vi "Dashboard Main.vi"() -> ()   [LabVIEW 2015]
uses:
  <vilib>/event_ctls.llb/eventvkey.ctl
  <vilib>/Utility/config.llb/NI_LVConfig.lvlib
  <vilib>/Rock Robotics/WPI/Dashboard/WPI_DashboardLogging Global.vi
  <vilib>/Utility/config.llb/Write Key (String).vi
  <vilib>/Utility/config.llb/Write Key (I32).vi
  TargetType.ctl
  <vilib>/Rock Robotics/WPI/Camera/WPI_CameraExposure Values.ctl
  <vilib>/Rock Robotics/WPI/Camera/WPI_CameraWhite Balance Values.ctl
panel:
  out "Image Message":string="Timeout in Camera Communications"
  in  "Rec Mode":enum32{"Stop", "Record", "Playback"}(radio)
  in  "Dashboard Tab":T1(tab)
  in  "Camera Settings":T2={"Frame Rate"=30, "Compression"=30, "Size"=1} {"Frame Rate" scale=1.0..30.0; "Size" items=["640x480", "320x240", "160x120"]}
  out "MotorSliders R":cluster{"MotorSlide1":dbl, "MotorSlide2":dbl} {"MotorSlide2" scale=-1.0..1.0 scale format="%#_2e"; "MotorSlide1" scale=-1.0..1.0 scale format="%#_2e"}
  out "MotorChart R":cluster{"Numeric":dbl, "Numeric":dbl}(graph)
  out "MotorSliders L":T3 {"MotorSlide4 2" scale=0.0..14.0 scale format="%#_2e"; "MotorSlide2" scale=-1.0..1.0 scale format="%#_2e"; "MotorSlide1" scale=-1.0..1.0 scale format="%#_2e"}
  out "MotorChart L":T4(graph)
  out "JS1 Z":dbl(slide) scale=-1.0..1.0 scale format="%#_2e"
  out "Joystick 1":cluster{"X":dbl, "Y":dbl}[](graph)
  out "JS Buttons 1":T5
  out "JS2 Z":dbl(slide) scale=-1.0..1.0 scale format="%#_2e"
  out "Joystick 2":cluster{"X":dbl, "Y":dbl}[](graph)
  out "JS Buttons 2":T5
  out "Mode":T6(ring)=enum."Auto Disabled"
  out "Camera IP":string
  in  "DB Camera Config":bool
  out "fps":dbl format="%#.1g"
  out "Mbps":dbl format="%#.1g"
  out "Mbps 2":bool
  out "LED 1":bool
  in  "Brightness":dbl(slide) scale=0.0..100.0
  in  "Color Level":dbl(slide) scale=0.0..100.0
  in  "Sharpness":dbl(slide) scale=0.0..100.0
  in  "Exposure":T7=enum."Hold current"
  in  "White Balance":T8
  in  "Move":T9(ring)=enum."Rook"
  in  "Score Limit":dbl=70.0
  in  "Color Components":T10={"Hue"={110.0, 142.0}, "Sat"={138.0, 255.0}, "Val"={139.0, 198.0}} {"Val" scale=0.0..255.0; "Sat" scale=0.0..255.0; "Hue" scale=0.0..255.0 scale format="%#_3g"}
  in  "Checkbox 2":bool
  in  "Checkbox 1":bool
  in  "Test Slider":dbl(slide) scale=0.0..100.0 scale format="%#_3g"
  in  "On/Off":bool caption="Solenoid"
  in  "Test Name":u16(ring) items=["Select the test to run...", "Example Test", "-------------------------------", "List of tests is built in robot code.", "Replace with your own automated tests."]
  in  "Test Tree":string(tree)
  in  "Motor":cluster{"Value":dbl, "Enable":bool} {"Value" scale=-1.0..1.0 scale format="%#_3g"}
  out "Progress":T11 {"Test Progress" scale=0.0..100.0}
  in  "Rev/Fwd":cluster{"Forward":bool, "Reverse":bool}
  in  "Test Ring":u16(ring) items=["Auto", "Fixed indoor", "Fixed outdoor 1", "Fixed outdoor 2", "Fixed fluorescent 1", "Fixed fluorescent 2", "Hold current"]
  in  "Listbox":i32(listbox)
  out "Tree":string(tree)
  out "Camera Image":T12(plugin-control)
  in  "Enable":bool=TRUE
  # "Left"
  # "Front"
  # "Right"
  # "Battery"
  # "This tab is a great place for autonomous settings and validation.\nCustomize by placing controls and indicators here and name to\nmatch Dashboard Variables on robot."
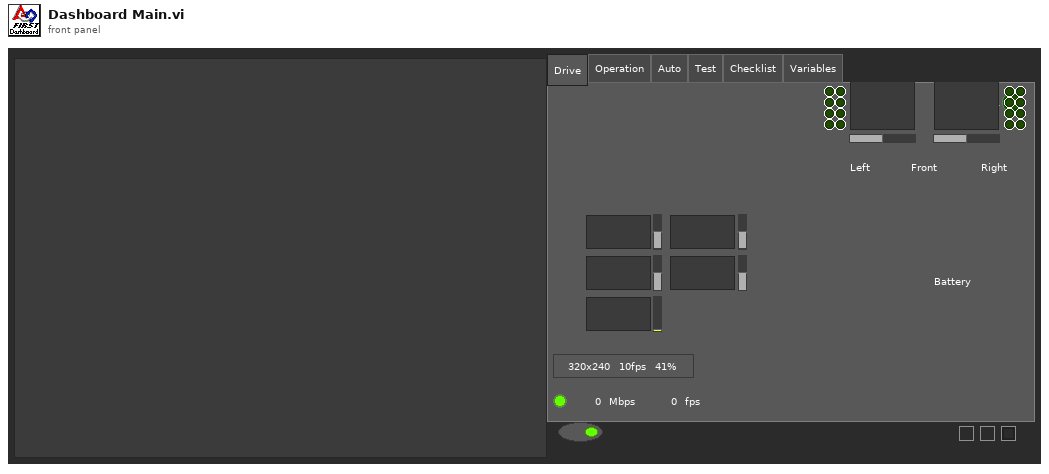
[diagram p1: front panel]
types:
  T1 = enum32{"Drive", "Operation", "Auto", "Test", "Checklist", "Variables"}
  T2 = cluster{"Frame Rate":i32, "Compression":i32, "Size":u16}
  T3 = cluster{"MotorSlide1":dbl, "MotorSlide2":dbl, "MotorSlide4 2":dbl}
  T4 = cluster{"Numeric":dbl, "Numeric":dbl, "Battery":sgl}
  T5 = cluster{bool, bool, bool, bool, bool, bool, bool, bool, bool, bool, bool, bool}
  T6 = enum8{"Tele-Op Disabled", "Tele-Op Enabled", "Auto Disabled", "Auto Enabled", "Test Disabled", "Test Enabled", ""}
  T7 = typedef "WPI_CameraExposure Values.ctl" = enum16{"Auto", "Flicker-free 50 Hz", "Flicker-free 60 Hz", "Hold current", "Custom"}
  T8 = typedef "WPI_CameraWhite Balance Values.ctl" = enum16{"Auto", "Fixed indoor", "Fixed outdoor 1", "Fixed outdoor 2", "Fixed fluorescent 1", "Fixed fluorescent 2", "Hold current", "Custom"}
  T9 = enum16{"Queen", "King", "Rook", "Knight", "Pawn"}
  T10 = cluster{"Hue":cluster{dbl, dbl}, "Sat":cluster{dbl, dbl}, "Val":cluster{dbl, dbl}}
  T11 = cluster{"Test Progress":u8, "Test Progress Text":string}
  T12 = typedef "IMAQ Image.ctl" = refnum<image>
  T13 = typedef "Image Type" = u32
  T14 = typedef "TargetType.ctl" = enum16{"Not Hot", "Hot"}
  T15 = cluster{"Horizontal":bool, "Aspect Score":dbl, "Rect Score":dbl, cluster{"Left":dbl, "Top":dbl, "Right":dbl, "Bottom":dbl}, "Equiv H":dbl, "Equiv V":dbl}[]
  T16 = cluster{"Scores":cluster{"Total":dbl, "Left":dbl, "Right":dbl, "Ratio":dbl, "Vertical":dbl, "index":i32, "State":T14}, "Verticals":cluster{"Horizontal?":bool, "Aspect Score":dbl, "Rect Score":dbl, cluster{"Left":dbl, "Top":dbl, "Right":dbl, "Bottom":dbl}, "Equiv H":dbl, "Equiv V":dbl}, "Horizontals":cluster{"Horizontal?":bool, "Aspect Score":dbl, "Rect Score":dbl, cluster{"Left":dbl, "Top":dbl, "Right":dbl, "Bottom":dbl}, "Equiv H":dbl, "Equiv V":dbl}, "Validated":bool}[]
  T17 = cluster{"Distance (ft)":dbl, "Target Center (-1 to 1)":cluster{"X":dbl, "Y":dbl}, "Left":bool, "State":T14, "Angle":dbl}[]
  T18 = cluster{cluster{dbl, dbl}, cluster{dbl, dbl}, cluster{dbl, dbl}}
  T19 = cluster{"Distance (ft)":dbl, "Target Center (-1 to 1)":cluster{"X":dbl, "Y":dbl}, "Left":bool, "State":T14, "Angle":dbl}
  T20 = cluster{"Digital Inputs":bool[], "Digital Outputs":bool[]}
  T21 = cluster{"Competition mode":bool, "Robot Link":bool, "Autonomous":bool, "Enabled":bool, "E-Stop":bool, "Simulated":bool, "TestMode":bool, "Docked Window":bool}
  T22 = cluster{"Boolean Array[0]":bool, "Boolean Array[1]":bool, "Boolean Array[2]":bool, "Boolean Array[3]":bool, "Boolean Array[4]":bool, "Boolean Array[5]":bool, "Boolean Array[6]":bool, "Boolean Array[7]":bool, "Boolean Array[8]":bool, "Boolean Array[9]":bool, "Boolean Array[10]":bool, "Boolean Array[11]":bool}
  T23 = typedef "NI_LVConfig.lvlib/Config Data RefNum.ctl" = refnum<k1>
  T24 = typedef "eventvkey.ctl" = enum16{"ASCII", "Enter", "Return", "Shift", "Ctrl", "Alt", "Cmd", "Opt", "Caps", "NumLock", "Clear", "Break", "Up", "Down", "Left", "Right", "Insert", "Delete", "Home", "End", "PageUp", "PageDown", "Escape", "Help", "Pause", "ScrollLock", "F1", "F2", "F3", "F4", "F5", "F6", "F7", "F8", "F9", "F10", "F11", "F12", "F13", "F14", "F15", "F16", "F17", "F18", "F19", "F20", "F21", "F22", "F23", "F24", "Play", "VolumeUp", "VolumeDown", "Mute", "Two Byte Char"}
  T25 = cluster{"Image Size":bool, "Image Type":bool, "Pixel Value":bool, "ROI Information":bool, "Zoom Factor":bool}
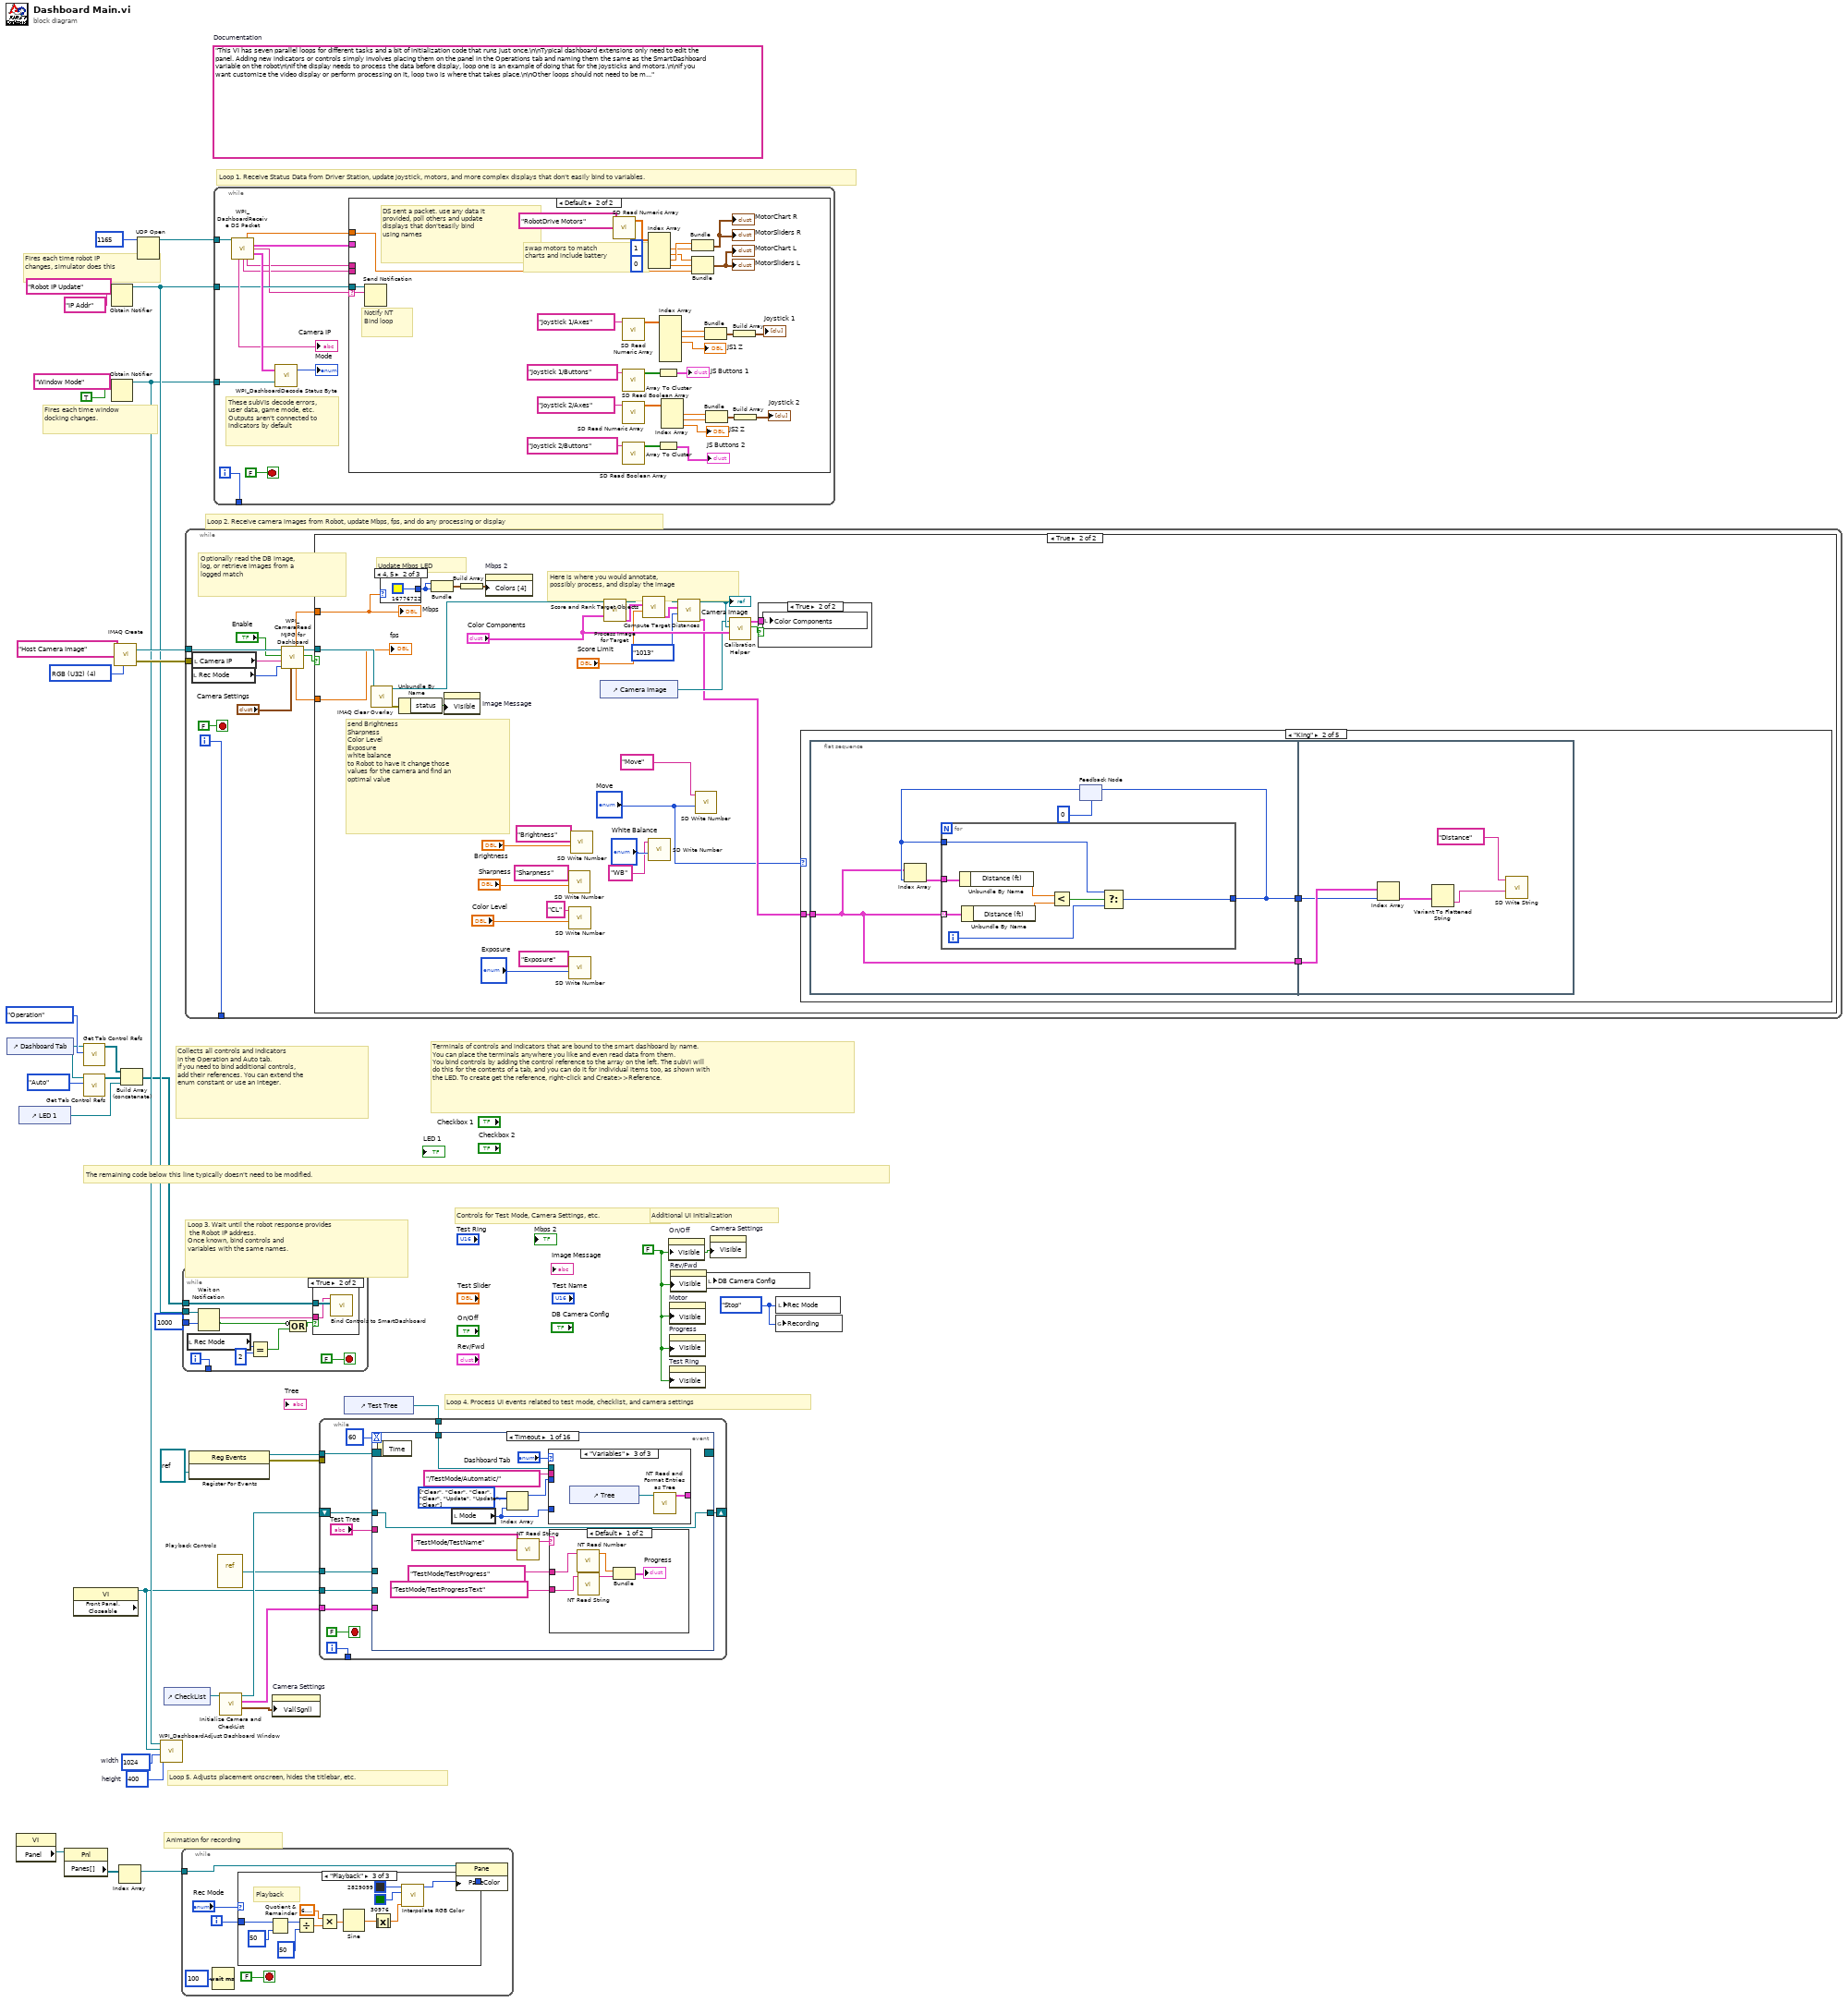
[diagram p0: block diagram]
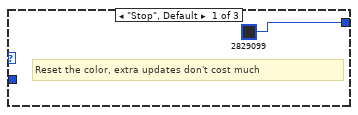
[diagram p2: hidden frame]
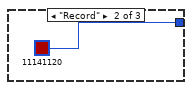
[diagram p3: hidden frame]
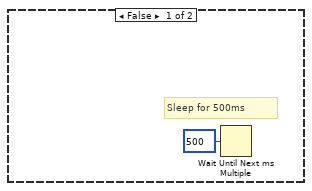
[diagram p5: hidden frame]
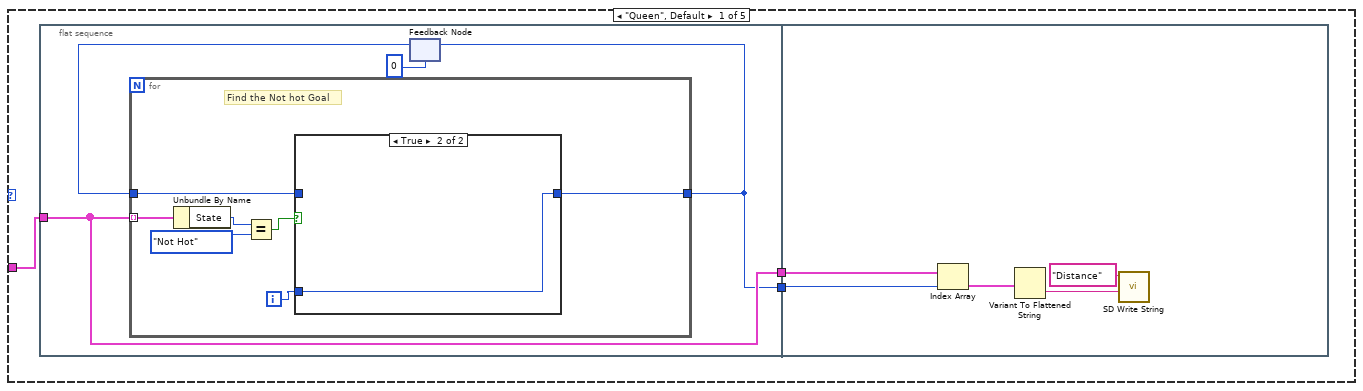
[diagram p6: hidden frame]
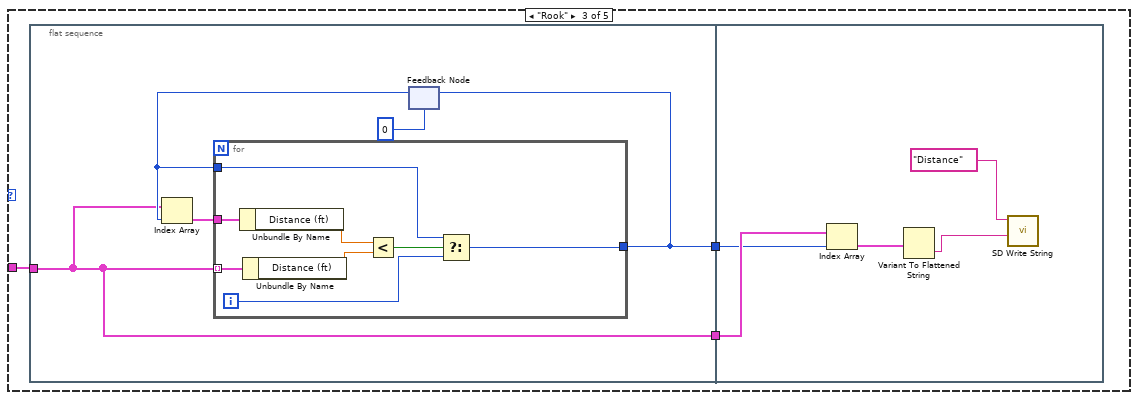
[diagram p8: hidden frame]
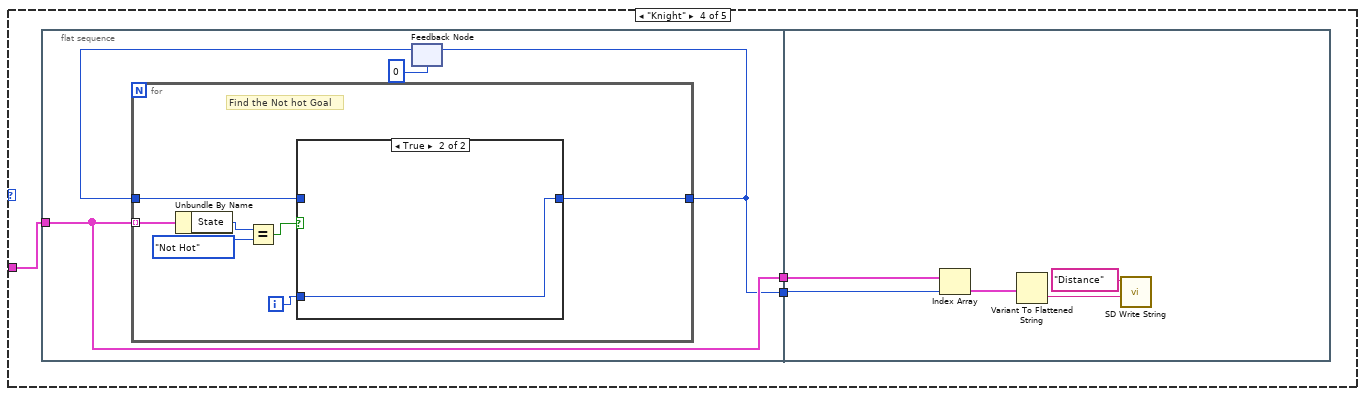
[diagram p9: hidden frame]
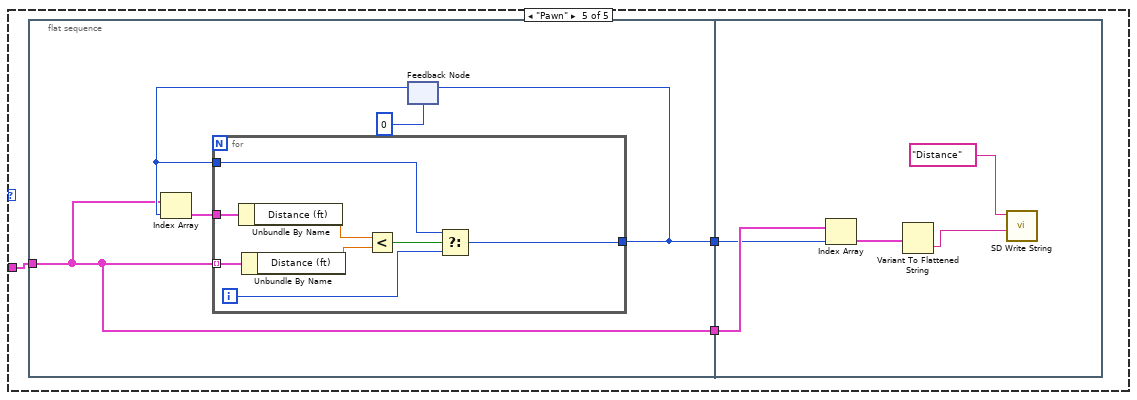
[diagram p11: hidden frame]
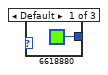
[diagram p13: hidden frame]
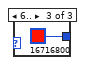
[diagram p14: hidden frame]
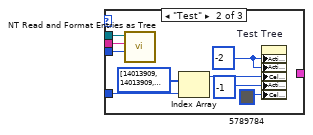
[diagram p16: hidden frame]
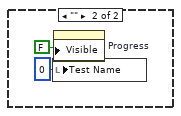
[diagram p17: hidden frame]
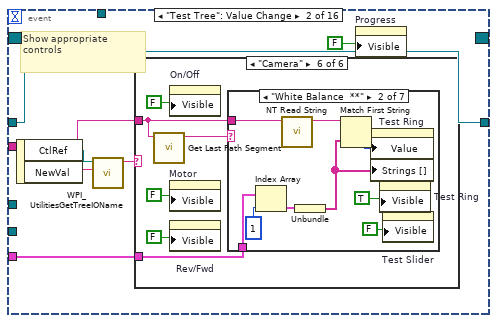
[diagram p18: hidden frame]
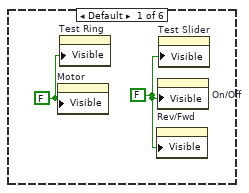
[diagram p19: hidden frame]
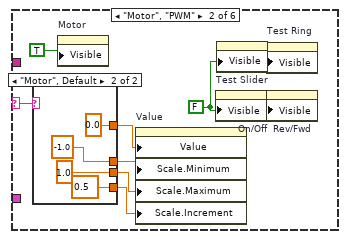
[diagram p20: hidden frame]
diagram:
  w8 = enum32{"Stop", "Record", "Playback"}."Stop" ("Rec Mode")
  w11 = 400  # height
  w12 = 1024  # width
  w25 = FALSE ("Visible")
  (unwired) "This VI has seven parallel loops for different tasks and a bit of initialization code that runs just once.\n\nTypical dashboard extensions only need to edit the panel. Adding new indicators or controls simply involves placing them on the panel in the Operations tab and naming them the same as the SmartDashboard variable on the robot\n\nIf the display needs to process the data before display, loop one is an example of doing that for the joysticks and motors.\n\nIf you want customize the video display or perform processing on it, loop two is where that takes place.\n\nOther loops should not need to be modified. They are pretty standard, and document the task they perform."  # Documentation
  w35 = T13 4 items=["Grayscale (U8)", "Grayscale (I16)", "Grayscale (SGL)", "Complex (CSG)", "RGB (U32)", "HSL (U32)", "RGB (U64)"] ("Image Type")
  # "Controls for Test Mode, Camera Settings, etc."
  # "Additional UI Initialization"
  # "Animation for recording"
  # "Fires each time robot IP\nchanges, simulator does this"
  # "Fires each time window\ndocking changes."
  # "Collects all controls and indicators\nin the Operation and Auto tab.\nIf you need to bind additional controls,\nadd their references. You can extend the\nenum constant or use an integer."
  # "The remaining code below this line typically doesn't need to be modified."
  # "Loop 4. Process UI events related to test mode, checklist, and camera settings"
  # "Terminals of controls and indicators that are bound to the smart dashboard by name.\nYou can place the terminals anywhere you like and even read data from them.\nYou bind controls by adding the control reference to the array on the left. The subVI will\ndo this for the contents of a tab, and you can do it for individual items too, as shown with\nthe LED. To create get the reference, right-click and Create>>Reference."
  # "Loop 3. Wait until the robot response provides\n the Robot IP address.\nOnce known, bind controls and\nvariables with the same names."
  # "Loop 5. Adjusts placement onscreen, hides the titlebar, etc."
  # "Loop 1. Receive Status Data from Driver Station, update joystick, motors, and more complex displays that don't easily bind to variables."
  # "Loop 2. Receive camera images from Robot, update Mbps, fps, and do any processing or display"
  n1 = control-ref of="Dashboard Tab"() -> (w6:refnum<vi>)
  n2 = property class="VI"() -> ("Panel"=w19:refnum<vi>)  [unwired: 2 in, 2 out]
  n3 = control-ref of="LED 1"() -> (w1:refnum<vi>)
  n4 = property class="Pnl"(reference=w19) -> ("Panes[]"=w20:refnum<vi>[])  [unwired: 1 in, 2 out]
  n5 = property class="VI" props=["Front Panel.Closeable"]() -> (reference out=w7:refnum<vi>)  [unwired: 2 in, 2 out]
  n6 = call <vilib>:"Get Tab Control Refs.vi"("Page Index"=T1."Operation" ("Dashboard Tab"), "TabControl in"=w6) -> ("ControlsOnPage"=w4:refnum<vi>[])  [unwired: 9 in]
  n7 = call <vilib>:"Get Tab Control Refs.vi"("Page Index"=T1."Auto" ("Dashboard Tab"), "TabControl in"=w6) -> ("ControlsOnPage"=w5:refnum<vi>[])  [unwired: 9 in]
  n8 = Obtain Notifier(name (unnamed)="Robot IP Update", notification data type="IP Addr" ("name (unnamed)")) -> (notifier out=w29:refnum<notifier>)  [unwired: 2 in, 2 out]
  n9 = Obtain Notifier(name (unnamed)="Window Mode", notification data type=TRUE) -> (notifier out=w10:refnum<notifier>)  [unwired: 2 in, 2 out]
  n10 = call "IMAQ Create"("Image Name"="Host Camera Image", "Image Type"=w35) -> ("New Image"=w33:T12, "error out"=w32:errorcluster)  [unwired: 2 in, 1 out]
  n11 = Index Array(array=w20) -> (element=w18:refnum<vi>)  [unwired: 1 in]
  n12 = Build Array (concatenate)(w4, w5, w1) -> (w3:refnum<vi>[])
  n13 = UDP Open(11:u16 1165 ("port")) -> (port=w36:refnum<k16>)  [unwired: 2 in, 4 out]
  n14 = call <vilib>:"WPI_DashboardAdjust Dashboard Window.vi"("height"=w11, "width"=w12, "reference in"=w7, "Notifier in"=w10) -> ()  [unwired: 8 in]
  n15 = control-ref of="CheckList"() -> (w9:refnum<vi>)
  n16 = while {
    tunnel: w18 -> [w39]
    i -> [w42]
    stop <- FALSE stop-if-true
    n17 = Wait (ms)(milliseconds to wait=u32 100) -> ()  [unwired: 1 out]
    n18 = case shown="\"Playback\"" "Rec Mode" {
      tunnel: w42 -> [_ _ w57]
      tunnel: [u32 2829099 ("Base Color") u32 11141120 ("Target Color") w46] -> w38
      frame "Stop", Default {
        # "Reset the color, extra updates don't cost much"
      }
      frame "Record" {
      }
      frame "Playback" {
        # "Playback"
        n19 = Quotient & Remainder(x=w57, y=u32 50 ("milliseconds to wait")) -> (x-y*floor(x/y)=w53:u32)  [unwired: 1 out]
        n20 = Divide(x=w53, y=u32 50 ("milliseconds to wait")) -> (x/y=w50:dbl)
        n21 = Multiply(x=6.283185307179586, y=w50) -> (x*y=w55:dbl)
        n22 = Sine(x=w55) -> (sin(x)=w54:dbl)
        n23 = Absolute Value(x=w54) -> (abs(x)=w47:dbl)
        n24 = call "Interpolate RGB Color.vi"("Proportion"=w47, "Target Color"=u32 30976, "Base Color"=u32 2829099) -> ("Result Color"=w46:u32)  [unwired: 8 in]
      }
    }
    n25 = property class="Pane"(reference=w39, "PaneColor"=w38) -> ()  [unwired: 1 in, 2 out]
  }
  n26 = while {
    tunnel: w3 -> [w68]
    tunnel: w29 -> [w66]
    tunnel: [w64] -> _
    tunnel: u32 1000 ("milliseconds to wait") -> [w63]
    i -> [w64]
    stop <- FALSE stop-if-true
    n27 = local read "Rec Mode"() -> (w59:enum32{"Stop", "Record", "Playback"})
    n28 = Wait on Notification(notifier=w66, timeout in ms (-1)=w63) -> (notification=w65:string, timed out?=w61:bool)  [unwired: 2 in, 2 out]
    n29 = Equal?(x=w59, y=u16 2 ("Rec Mode")) -> (x = y?=w60:bool)
    n30 = Compound Arithmetic op=OR(invert w61, w60) -> (w62:bool)
    n31 = case shown="True" w62 {
      tunnel: w68 -> [_ w70]
      tunnel: w65 -> [_ w69]
      frame False {
      }
      frame True {
        n32 = call <vilib>:"Bind Controls to SmartDashboard.vi"("Bound Control Refs"=w70, "Server IP Address"=w69) -> ()  [unwired: 10 in]
      }
    }
  }
  n33 = while {
    tunnel: w33 -> [w79]
    tunnel: w32 -> [_]
    tunnel: [w80] -> _
    i -> [w80]
    stop <- FALSE stop-if-true
    # "Optionally read the DB image,\nlog, or retrieve images from a\nlogged match"
    n34 = local read "Rec Mode"() -> (w71:enum32{"Stop", "Record", "Playback"})
    n35 = local read "Camera IP"() -> (w72:string)
    n36 = call <vilib>:"WPI_CameraRead MJPG for Dashboard.vi"("Camera Settings"="Camera Settings", "Rec Mode"=w71, "Camera IP"=w72, "Camera Mode"="Enable", "Refnum in"=w79) -> ("Active"=w76:bool, "Refnum out"=w78:T12, "FPS"=w75:dbl, "Bandwidth (Mbps)"=w74:dbl)  [unwired: 3 in]
    n37 = case shown="True" w76 {
      tunnel: w78 -> [_ w110]
      tunnel: w74 -> [_ w109]
      tunnel: w75 -> [_ w108]
      frame False {
        # "Sleep for 500ms"
        n38 = Wait Until Next ms Multiple(millisecond multiple=u32 500) -> ()  [unwired: 1 out]
      }
      frame True {
        # "send Brightness\nSharpness\nColor Level\nExposure\nwhite balance\nto Robot to have it change those\nvalues for the camera and find an \noptimal value"
        # "Here is where you would annotate,\npossibly process, and display the image"
        # "Update Mbps LED"
        n39 = call "IMAQ Clear Overlay"("Image"=w110) -> ("error out"=w114:errorcluster, "Image Out"=w107:T12)  [unwired: 2 in, 7 out]
        n40 = case shown="4, 5" w109 {
          tunnel: [u32 6618880 ("Color Box") u32 16776722 ("Color Box") u32 16716800 ("Color Box")] -> w111
          frame Default {
          }
          frame 4, 5 {
          }
          frame 6.. {
          }
        }
        n41 = Unbundle By Name(w114) -> ("status"=w115:bool)
        n42 = Bundle("Color Box"=w111, "Color Box"=w111) -> (w113:cluster{"Color Box":u32, "Color Box":u32})  [unwired: 1 out]
        n43 = property on="Image Message" class="Str"("Visible"=w115) -> ()  [unwired: 2 in, 2 out]
        n44 = Build Array(w113) -> (w112:cluster{"Color Box":u32, "Color Box":u32}[])
        n45 = property on="Mbps 2" class="Bool (strict)"("Colors [4]"=w112) -> ()  [unwired: 2 in, 2 out]
        n46 = call <vilib>:"SD Write Number.vi"("Numeric"="Sharpness", "Name"="Sharpness") -> ()  [unwired: 8 in, 2 out]
        n47 = call <vilib>:"SD Write Number.vi"("Numeric"="Color Level", "Name"="CL") -> ()  [unwired: 8 in, 2 out]
        n48 = call <vilib>:"SD Write Number.vi"("Numeric"="Exposure", "Name"="Exposure") -> ()  [unwired: 8 in, 2 out]
        n49 = call <vilib>:"SD Write Number.vi"("Numeric"="Brightness", "Name"="Brightness") -> ()  [unwired: 8 in, 2 out]
        n50 = control-ref of="Camera Image"() -> (w97:refnum<vi>)
        n51 = call "Process Image for Target.vi"("Src Image"=w107, "Color Components"="Color Components") -> ("Src Image Out"=w106:T12, "Particles"=w99:T15)  [unwired: 11 in, 1 out]
        n52 = call "Score and Rank Target Objects.vi"("Score Limit"="Score Limit", "Particles"=w99, "Image in"=w106) -> ("Target Info"=w98:T16, "Annotated Image"=w105:T12)  [unwired: 7 in]
        n53 = call <vilib>:"SD Write Number.vi"("Numeric"="White Balance", "Name"="WB") -> ()  [unwired: 8 in, 2 out]
        n54 = call "Compute Target Distances.vi"("Camera Type"=enum16{"206", "1011", "1013"}."1013", "Target Info"=w98, "Image in"=w105) -> ("Distances"=w95:T17, "Image out"=w104:T12)  [unwired: 6 in, 1 out]
        "Camera Image" <- w104
        n55 = call <vilib>:"SD Write Number.vi"("Numeric"="Move", "Name"="Move") -> ()  [unwired: 8 in, 2 out]
        n56 = call "Calibration Helper.vi"("Color Components"="Color Components", "Image"=w104, "Image Ctl Refnum"=w97) -> ("Changed"=w96:bool, "output color"=w102:T18)  [unwired: 7 in]
        n57 = case shown="True" w96 {
          tunnel: w102 -> [_ w221]
          frame False {
          }
          frame True {
            n58 = local write "Color Components"(w221) -> ()
          }
        }
        n59 = case shown="\"King\"" "Move" {
          tunnel: w95 -> [w118 w137 w158 w179 w200]
          frame "Queen", Default {
            n60 = flat-sequence {
              tunnel: w118 -> [w120]
              tunnel: [w120] -> w117
              tunnel: [w119] -> w116
              tunnel: w117 -> [w133]
              tunnel: w116 -> [w132]
              frame #0 {
                n61 = feedback #1(0) -> (w122:i32)
                n62 = for {
                  tunnel: w120 -> [w129] mode=indexing
                  tunnel: [w123] -> w119
                  tunnel: w122 -> [w124]
                  i -> [w125]
                  # "Find the Not hot Goal"
                  n63 = Unbundle By Name(w129) -> ("State"=w128:T14)
                  n64 = Equal?(x=w128, y=TargetType."Not Hot" ("State")) -> (x = y?=w126:bool)
                  n65 = case shown="True" w126 {
                    tunnel: w125 -> [_ w131]
                    tunnel: w124 -> [w130 _]
                    tunnel: [w130 w131] -> w123
                    frame False {
                    }
                    frame True {
                    }
                  }
                }
                n66 = feedback-in #1(w119) -> ()
              }
              frame #1 {
                n67 = Index Array(array=w133, index=w132) -> (element=w134:T19)
                n68 = Variant To Flattened String(Variant=w134) -> (data string=w135:string)  [unwired: 1 out]
                n69 = call <vilib>:"SD Write String.vi"("String"=w135, "Name"="Distance") -> ()  [unwired: 8 in, 2 out]
              }
            }
          }
          frame "King" {
            n70 = flat-sequence {
              tunnel: w137 -> [w141]
              tunnel: [w141] -> w139
              tunnel: [w140] -> w138
              tunnel: w139 -> [w157]
              tunnel: w138 -> [w156]
              frame #0 {
                n71 = feedback #2(0) -> (w142:i32)
                n72 = Index Array(array=w141, index=w142) -> (element=w143:T19)
                n73 = for {
                  tunnel: w141 -> [w152] mode=indexing
                  tunnel: [w145] -> w140
                  tunnel: w143 -> [w150]
                  tunnel: w142 -> [w146]
                  i -> [w147]
                  n74 = Unbundle By Name(w150) -> ("Distance (ft)"=w149:dbl)
                  n75 = Unbundle By Name(w152) -> ("Distance (ft)"=w151:dbl)
                  n76 = Less?(x=w149, y=w151) -> (x < y?=w148:bool)
                  n77 = Select(t=w146, s=w148, f=w147) -> (s? t:f=w145:i32)
                }
                n78 = feedback-in #2(w140) -> ()
              }
              frame #1 {
                n79 = Index Array(array=w157, index=w156) -> (element=w153:T19)
                n80 = Variant To Flattened String(Variant=w153) -> (data string=w154:string)  [unwired: 1 out]
                n81 = call <vilib>:"SD Write String.vi"("String"=w154, "Name"="Distance") -> ()  [unwired: 8 in, 2 out]
              }
            }
          }
          frame "Rook" {
            n82 = flat-sequence {
              tunnel: w158 -> [w162]
              tunnel: [w162] -> w160
              tunnel: [w161] -> w159
              tunnel: w160 -> [w178]
              tunnel: w159 -> [w177]
              frame #0 {
                n83 = feedback #3(0) -> (w163:i32)
                n84 = Index Array(array=w162, index=w163) -> (element=w164:T19)
                n85 = for {
                  tunnel: w162 -> [w173] mode=indexing
                  tunnel: [w166] -> w161
                  tunnel: w164 -> [w171]
                  tunnel: w163 -> [w167]
                  i -> [w168]
                  n86 = Unbundle By Name(w171) -> ("Distance (ft)"=w170:dbl)
                  n87 = Unbundle By Name(w173) -> ("Distance (ft)"=w172:dbl)
                  n88 = Less?(x=w170, y=w172) -> (x < y?=w169:bool)
                  n89 = Select(t=w167, s=w169, f=w168) -> (s? t:f=w166:i32)
                }
                n90 = feedback-in #3(w161) -> ()
              }
              frame #1 {
                n91 = Index Array(array=w178, index=w177) -> (element=w174:T19)
                n92 = Variant To Flattened String(Variant=w174) -> (data string=w175:string)  [unwired: 1 out]
                n93 = call <vilib>:"SD Write String.vi"("String"=w175, "Name"="Distance") -> ()  [unwired: 8 in, 2 out]
              }
            }
          }
          frame "Knight" {
            n94 = flat-sequence {
              tunnel: w179 -> [w183]
              tunnel: [w183] -> w181
              tunnel: [w182] -> w180
              tunnel: w181 -> [w196]
              tunnel: w180 -> [w195]
              frame #0 {
                n95 = feedback #4(0) -> (w185:i32)
                n96 = for {
                  tunnel: w183 -> [w192] mode=indexing
                  tunnel: [w186] -> w182
                  tunnel: w185 -> [w187]
                  i -> [w188]
                  # "Find the Not hot Goal"
                  n97 = Unbundle By Name(w192) -> ("State"=w191:T14)
                  n98 = Equal?(x=w191, y=TargetType."Not Hot" ("State")) -> (x = y?=w189:bool)
                  n99 = case shown="True" w189 {
                    tunnel: w188 -> [_ w194]
                    tunnel: w187 -> [w193 _]
                    tunnel: [w193 w194] -> w186
                    frame False {
                    }
                    frame True {
                    }
                  }
                }
                n100 = feedback-in #4(w182) -> ()
              }
              frame #1 {
                n101 = Index Array(array=w196, index=w195) -> (element=w197:T19)
                n102 = Variant To Flattened String(Variant=w197) -> (data string=w198:string)  [unwired: 1 out]
                n103 = call <vilib>:"SD Write String.vi"("String"=w198, "Name"="Distance") -> ()  [unwired: 8 in, 2 out]
              }
            }
          }
          frame "Pawn" {
            n104 = flat-sequence {
              tunnel: w200 -> [w204]
              tunnel: [w204] -> w202
              tunnel: [w203] -> w201
              tunnel: w202 -> [w220]
              tunnel: w201 -> [w219]
              frame #0 {
                n105 = feedback #5(0) -> (w205:i32)
                n106 = Index Array(array=w204, index=w205) -> (element=w206:T19)
                n107 = for {
                  tunnel: w204 -> [w215] mode=indexing
                  tunnel: [w208] -> w203
                  tunnel: w206 -> [w213]
                  tunnel: w205 -> [w209]
                  i -> [w210]
                  n108 = Unbundle By Name(w213) -> ("Distance (ft)"=w212:dbl)
                  n109 = Unbundle By Name(w215) -> ("Distance (ft)"=w214:dbl)
                  n110 = Less?(x=w212, y=w214) -> (x < y?=w211:bool)
                  n111 = Select(t=w209, s=w211, f=w210) -> (s? t:f=w208:i32)
                }
                n112 = feedback-in #5(w203) -> ()
              }
              frame #1 {
                n113 = Index Array(array=w220, index=w219) -> (element=w216:T19)
                n114 = Variant To Flattened String(Variant=w216) -> (data string=w217:string)  [unwired: 1 out]
                n115 = call <vilib>:"SD Write String.vi"("String"=w217, "Name"="Distance") -> ()  [unwired: 8 in, 2 out]
              }
            }
          }
        }
        "Mbps" <- w109
        "fps" <- w108
      }
    }
  }
  n116 = register-events(refnum<vi> refnum) -> (reference out=w16:refnum<event-registration>, error out=w15:errorcluster)  [unwired: 2 in]
  n117 = while {
    tunnel: w36 -> [w235]
    tunnel: w29 -> [w230]
    tunnel: w10 -> [w234]
    tunnel: [w231] -> _
    i -> [w231]
    stop <- FALSE stop-if-true
    # "These subVIs decode errors, user data, game mode, etc.\nOutputs aren't connected to indicators by default"
    n118 = call <vilib>:"WPI_DashboardReceive DS Packet.vi"("Recv Socket"=w235) -> ("Battery"=w225:sgl, "Driver Station"=w226:T20, "Robot IP Address"=w229:string, "Status"=w236:T21, "Camera IP Address"=→"Camera IP":string, "Low Priority User Data"=w228:string, "High Priority User Data"=w227:string)  [unwired: 2 in, 6 out]
    n119 = call <vilib>:"WPI_DashboardDecode Status Byte.vi"("Window Mode Notifier"=w234, "Status"=w236) -> ("Mode"=→"Mode":T6)  [unwired: 1 out]
    n120 = case shown="Default" w229 {
      selector: w229 -> [_ w248]
      tunnel: w230 -> [_ w249]
      tunnel: w228 -> [_ _]
      tunnel: w227 -> [_ _]
      tunnel: w226 -> [_ _]
      tunnel: w225 -> [_ w247]
      frame "0.0.0.0" {
        # "DS not sending packets, or no robot exists yet.\nDon't poll the variables"
      }
      frame Default {
        # "Notify NT\nBind loop"
        # "DS sent a packet. use any data it\nprovided, poll others and update\ndisplays that don'teasily bind\nusing names"
        # "swap motors to match\ncharts and include battery"
        n121 = Send Notification(notification=w248, notifier=w249) -> ()  [unwired: 1 in, 2 out]
        n122 = call <vilib>:"SD Read Numeric Array.vi"("Name"="RobotDrive Motors") -> ("Numeric Array"=w246:dbl[])  [unwired: 8 in, 2 out]
        n123 = call <vilib>:"SD Read Numeric Array.vi"("Name"="Joystick 1/Axes") -> ("Numeric Array"=w265:dbl[])  [unwired: 8 in, 2 out]
        n124 = call <vilib>:"SD Read Boolean Array.vi"("Name"="Joystick 1/Buttons") -> ("Boolean Array"=w267:bool[])  [unwired: 8 in, 2 out]
        n125 = call <vilib>:"SD Read Numeric Array.vi"("Name"="Joystick 2/Axes") -> ("Numeric Array"=w259:dbl[])  [unwired: 8 in, 2 out]
        n126 = call <vilib>:"SD Read Boolean Array.vi"("Name"="Joystick 2/Buttons") -> ("Boolean Array"=w258:bool[])  [unwired: 8 in, 2 out]
        n127 = Index Array(array=w246, index #1=1, index #4=0) -> (element #1=w242:dbl, element #2=w241:dbl, element #3=w243:dbl, element #4=w238:dbl)  [unwired: 2 in]
        n128 = Array To Cluster(array=w267) -> (cluster=→"JS Buttons 1":T22)
        n129 = Array To Cluster(array=w258) -> (cluster=→"JS Buttons 2":T22)
        n130 = Index Array(array=w265) -> (element #1=w262:dbl, element #2=w263:dbl, element #3=→"JS1 Z":dbl)  [unwired: 6 in, 3 out]
        n131 = Index Array(array=w259) -> (element #1=w254:dbl, element #2=w253:dbl, element #3=→"JS2 Z":dbl)  [unwired: 3 in]
        n132 = Bundle("Numeric"=w243, "Numeric"=w242) -> (→"MotorChart R" →"MotorSliders R":cluster{"Numeric":dbl, "Numeric":dbl})  [unwired: 1 in]
        n133 = Bundle("Numeric"=w241, "Numeric"=w238, "Battery"=w247) -> (→"MotorChart L" →"MotorSliders L":T4)  [unwired: 1 in]
        n134 = Bundle("Numeric"=w262, "Numeric"=w263) -> (w261:cluster{"Numeric":dbl, "Numeric":dbl})  [unwired: 1 in]
        n135 = Bundle("Numeric"=w254, "Numeric"=w253) -> (w255:cluster{"Numeric":dbl, "Numeric":dbl})  [unwired: 1 in]
        n136 = Build Array(w261) -> (→"Joystick 1":cluster{"Numeric":dbl, "Numeric":dbl}[])
        n137 = Build Array(w255) -> (→"Joystick 2":cluster{"Numeric":dbl, "Numeric":dbl}[])
      }
    }
  }
  n138 = vi-ref "Playback Controls.vi"() -> (w17:refnum<vi>)
  n139 = call "Initialize Camera and CheckList.vi"("ListBox in"=w9) -> ("Cluster"=w23:cluster{"value":i32, "value":i32, "index":i32}, "Array"=w24:cluster{string[]}[], "File Refnum"=w22:T23)  [unwired: 8 in]
  n140 = property on="Camera Settings" class="Clust (strict)"("Val(Sgnl)"=w23) -> ()  [unwired: 2 in, 2 out]
  n141 = control-ref of="Test Tree"() -> (w21:refnum<vi>)
  n142 = while {
    tunnel: w24 -> [w278]
    shift-right: [w277] -> _
    shift-left: w22 -> [w276]
    tunnel: [w275] -> _
    tunnel: w21 -> [w274]
    tunnel: w17 -> [w273]
    tunnel: w16 -> [w272]
    tunnel: w15 -> [_]
    tunnel: w7 -> [w271]
    i -> [w275]
    stop <- FALSE stop-if-true
    n143 = event shown="[0] Timeout" {
      selector: w272 -> [_ _ _ _ _ _ _ _ _ _ _ _ _ _ _ _]
      dyn-events: [_ _ _ _ _ _ _ _ _ _ _ _ _ w516 _ _] -> _
      timeout: u32 60 ("milliseconds to wait") -> [_ _ _ _ _ _ _ _ _ _ _ _ _ _ _ _]
      tunnel: w274 -> [w288 _ _ _ _ _ _ _ _ _ _ _ _ _ _ _]
      tunnel: "Test Tree" -> [_ _ _ _ _ _ _ _ w485 w493 w495 w499 w507 _ _ _]
      tunnel: w278 -> [_ w312 _ _ _ _ w449 w479 _ _ _ _ _ _ _ _]
      tunnel: [w282 w311 w410 w415 w423 w435 w448 w472 w484 w491 w494 w498 w506 w518 w532 w533] -> w277
      tunnel: w276 -> [w282 w311 w410 w415 w423 w435 w447 w472 w484 w491 w494 w498 w506 w518 w532 w533]
      tunnel: w273 -> [_ _ _ _ _ _ _ _ _ _ _ _ _ w519 _ w536]
      tunnel: w271 -> [_ _ _ _ _ _ _ _ _ _ _ _ _ w514 _ _]
      event Timeout {
        w287 = enum16{"Update", "Clear"}[] [enum."Clear", enum."Clear", enum."Clear", enum."Clear", enum."Update", enum."Update", enum."Clear"] items=["Update", "Clear"]
        n144 = event-data() -> ()  [unwired: 1 in, 1 out]
        n145 = local read "Mode"() -> (w285:T6)
        n146 = Index Array(array=w287, index=w285) -> (element=w286:enum16{"Update", "Clear"})
        n147 = call <vilib>:"NT Read String.vi"("Name"="TestMode/TestName") -> ("String"=w291:string)  [unwired: 9 in, 1 out]
        n148 = case shown="\"Variables\"" "Dashboard Tab" {
          tunnel: w288 -> [_ w301 _]
          tunnel: "/TestMode/Automatic/" ("Name Pattern") -> [_ w300 _]
          tunnel: w286 -> [_ w299 _]
          tunnel: w285 -> [_ w297 _]
          tunnel: [_ _ w303] -> _
          frame "Operation", Default {
          }
          frame "Test" {
            w296 = -2 ("Active Item:Row Number")
            n149 = call <vilib>:"NT Read and Format Entries as Tree.vi"("Operation"=w299, "Name Pattern"=w300, "Tree Refnum"=w301) -> ()  [unwired: 7 in, 2 out]
            n150 = Index Array(array=u32[] [14013909, 14013909, 14013909, 14013909, 14013909, 16777215, 14013909], index=w297) -> (element=w295:u32)
            n151 = property on="Test Tree" class="Tree (strict)"("Active Item Row Number"=w296, "ActiveColNum"=w296, "CellBG"=w295, "Active Item Row Number"=-1 ("Active Item:Row Number"), "CellBG"=u32 5789784 ("Color Box")) -> ()  [unwired: 2 in, 2 out]
          }
          frame "Variables" {
            n152 = control-ref of="Tree"() -> (w302:refnum<vi>)
            n153 = call <vilib>:"NT Read and Format Entries as Tree.vi"("Tree Refnum"=w302) -> ("Formatted Strings"=w303:cluster{"Name":string, "Value":string}[])  [unwired: 9 in, 1 out]
          }
        }
        n154 = case shown="Default" w291 {
          tunnel: "TestMode/TestProgress" ("Name") -> [w305 _]
          tunnel: "TestMode/TestProgressText" ("Name") -> [w304 _]
          frame Default {
            n155 = call <vilib>:"NT Read Number.vi"("Name"=w305) -> ("Numeric"=w306:dbl)  [unwired: 9 in, 1 out]
            n156 = call <vilib>:"NT Read String.vi"("Name"=w304) -> ("String"=w307:string)  [unwired: 9 in, 1 out]
            n157 = Bundle("Numeric"=w306, "String"=w307) -> (→"Progress":cluster{"Numeric":dbl, "String":string})  [unwired: 1 in]
          }
          frame "" {
            n158 = local write "Test Name"(u16 0) -> ()
            n159 = property on="Progress" class="Clust (strict)"("Visible"=FALSE) -> ()  [unwired: 2 in, 2 out]
          }
        }
      }
      event "Test Tree": Value Change {
        # "Show appropriate\ncontrols"
        n160 = event-data() -> ("CtlRef"=w315:refnum<vi>, "NewVal"=w313:string)  [unwired: 1 in]
        n161 = call <vilib>:"WPI_UtilitiesGetTreeIOName.vi"("NewVal"=w313, "TreeControl in"=w315) -> ("I/O Name"=w316:string)  [unwired: 9 in]
        n162 = case shown="\"Camera\"" w316 {
          selector: w316 -> [_ w323 _ w341 w350 _]
          tunnel: w313 -> [_ _ w338 w340 _ w357]
          tunnel: w312 -> [_ _ _ _ _ w356]
          frame Default {
            w318 = FALSE ("Visible")
            w317 = FALSE ("Visible")
            n163 = property on="Motor" class="Clust (strict)"("Visible"=w317) -> ()  [unwired: 2 in, 2 out]
            n164 = property on="Test Ring" class="Ring (strict)"("Visible"=w317) -> ()  [unwired: 2 in, 2 out]
            n165 = property on="Rev/Fwd" class="Clust (strict)"("Visible"=w318) -> ()  [unwired: 2 in, 2 out]
            n166 = property on="On/Off" class="Bool (strict)"("Visible"=w318) -> ()  [unwired: 2 in, 2 out]
            n167 = property on="Test Slider" class="Slide (strict)"("Visible"=w318) -> ()  [unwired: 2 in, 2 out]
          }
          frame "Motor", "PWM" {
            w324 = FALSE ("Visible")
            n168 = case shown="\"Motor\", Default" w323 {
              tunnel: [1.0 ("Value") -1.0 ("Value")] -> w322
              tunnel: [255.0 ("Value") 1.0 ("Value")] -> w321
              tunnel: [128.0 ("Value") 0.0 ("Value")] -> w320
              tunnel: [64.0 ("Value") 0.5 ("Value")] -> w319
              frame "PWM" {
              }
              frame "Motor", Default {
              }
            }
            n169 = property on="Motor" class="Clust (strict)"("Visible"=TRUE) -> ()  [unwired: 2 in, 2 out]
            n170 = property on="Value" class="Slide (strict)"("Value"=w320, "Scale.Minimum"=w322, "Scale.Maximum"=w321, "Scale.Increment"=w319) -> ()  [unwired: 2 in, 2 out]
            n171 = property on="On/Off" class="Bool (strict)"("Visible"=w324) -> ()  [unwired: 2 in, 2 out]
            n172 = property on="Test Slider" class="Slide (strict)"("Visible"=w324) -> ()  [unwired: 2 in, 2 out]
            n173 = property on="Test Ring" class="Ring (strict)"("Visible"=w324) -> ()  [unwired: 2 in, 2 out]
            n174 = property on="Rev/Fwd" class="Clust (strict)"("Visible"=w324) -> ()  [unwired: 2 in, 2 out]
          }
          frame "Servo" {
            w336 = FALSE ("Visible")
            n175 = call <vilib>:"NT Read Number.vi"("Name"=w338) -> ("Numeric"=w337:dbl)  [unwired: 9 in, 1 out]
            n176 = property on="Test Slider" class="Slide (strict)"("Visible"=TRUE, "Scale.Maximum"=170.0 ("Scale.Range:Maximum")) -> ()  [unwired: 2 in, 2 out]
            n177 = local write "Test Slider"(w337) -> ()
            n178 = property on="Motor" class="Clust (strict)"("Visible"=w336) -> ()  [unwired: 2 in, 2 out]
            n179 = property on="Rev/Fwd" class="Clust (strict)"("Visible"=w336) -> ()  [unwired: 2 in, 2 out]
            n180 = property on="On/Off" class="Bool (strict)"("Visible"=w336) -> ()  [unwired: 2 in, 2 out]
            n181 = property on="Test Ring" class="Ring (strict)"("Visible"=w336) -> ()  [unwired: 2 in, 2 out]
          }
          frame "Relay", "Solenoid" {
            w339 = FALSE ("Visible")
            n182 = property on="Motor" class="Clust (strict)"("Visible"=w339) -> ()  [unwired: 2 in, 2 out]
            n183 = property on="Test Slider" class="Slide (strict)"("Visible"=w339) -> ()  [unwired: 2 in, 2 out]
            n184 = Search and Replace String(input string=w340, search string="/Value  **", replace string="/Direction") -> (result string=w346:string)  [unwired: 5 in, 3 out]
            n185 = property on="Test Ring" class="Ring (strict)"("Visible"=w339) -> ()  [unwired: 2 in, 2 out]
            n186 = call <vilib>:"NT Read String.vi"("Name"=w346) -> ("String"=w344:string)  [unwired: 9 in, 1 out]
            n187 = Equal?(x="Both directions", y=w344) -> (x = y?=w342:bool)
            n188 = Not(x=w342) -> (.not. x?=w343:bool)
            n189 = property on="Rev/Fwd" class="Clust (strict)"("Visible"=w342) -> ()  [unwired: 2 in, 2 out]
            n190 = property on="On/Off" class="Bool (strict)"("Visible"=w343, "Caption.Text"=w341) -> ()  [unwired: 2 in, 2 out]
          }
          frame "Compressor", "Digital Out" {
            w349 = FALSE ("Visible")
            # "Get direction and finish"
            n191 = property on="Motor" class="Clust (strict)"("Visible"=w349) -> ()  [unwired: 2 in, 2 out]
            n192 = property on="Test Slider" class="Slide (strict)"("Visible"=w349) -> ()  [unwired: 2 in, 2 out]
            n193 = property on="Test Ring" class="Ring (strict)"("Visible"=w349) -> ()  [unwired: 2 in, 2 out]
            n194 = property on="On/Off" class="Bool (strict)"("Visible"=TRUE, "Caption.Text"=w350) -> ()  [unwired: 2 in, 2 out]
            n195 = property on="Rev/Fwd" class="Clust (strict)"("Visible"=FALSE) -> ()  [unwired: 2 in, 2 out]
          }
          frame "Camera" {
            n196 = call <vilib>:"Get Last Path Segment.vi"("String in"=w357) -> ("String out"=w358:string)  [unwired: 10 in]
            n197 = property on="On/Off" class="Bool (strict)"("Visible"=FALSE) -> ()  [unwired: 2 in, 2 out]
            n198 = property on="Motor" class="Clust (strict)"("Visible"=FALSE) -> ()  [unwired: 2 in, 2 out]
            n199 = property on="Rev/Fwd" class="Clust (strict)"("Visible"=FALSE) -> ()  [unwired: 2 in, 2 out]
            n200 = case shown="\"White Balance  **\"" w358 {
              tunnel: w357 -> [w364 w373 w382 w391 w400 _ w406]
              tunnel: w356 -> [w362 w370 w379 w388 w397 _ _]
              frame "Size  **" {
                n201 = Index Array(array=w362) -> (element=w361:cluster{string[]})  [unwired: 1 in]
                n202 = call <vilib>:"NT Read String.vi"("Name"=w364) -> ("String"=w363:string)  [unwired: 9 in, 1 out]
                n203 = Unbundle(w361) -> (w359:string[])
                n204 = Match First String(2:w359, 3:w363) -> (0:w360:i32)  [unwired: 1 out]
                n205 = property on="Test Ring" class="Ring (strict)"("Value"=w360, "Strings []"=w359) -> ()  [unwired: 2 in, 2 out]
                n206 = property on="Test Ring" class="Ring (strict)"("Visible"=TRUE) -> ()  [unwired: 2 in, 2 out]
                n207 = property on="Test Slider" class="Slide (strict)"("Visible"=FALSE) -> ()  [unwired: 2 in, 2 out]
              }
              frame "White Balance  **" {
                n208 = Index Array(array=w370, index=1) -> (element=w371:cluster{string[]})
                n209 = call <vilib>:"NT Read String.vi"("Name"=w373) -> ("String"=w372:string)  [unwired: 9 in, 1 out]
                n210 = Unbundle(w371) -> (w368:string[])
                n211 = Match First String(2:w368, 3:w372) -> (0:w367:i32)  [unwired: 1 out]
                n212 = property on="Test Ring" class="Ring (strict)"("Value"=w367, "Strings []"=w368) -> ()  [unwired: 2 in, 2 out]
                n213 = property on="Test Ring" class="Ring (strict)"("Visible"=TRUE) -> ()  [unwired: 2 in, 2 out]
                n214 = property on="Test Slider" class="Slide (strict)"("Visible"=FALSE) -> ()  [unwired: 2 in, 2 out]
              }
              frame "Exposure  **" {
                n215 = Index Array(array=w379, index=2) -> (element=w380:cluster{string[]})
                n216 = call <vilib>:"NT Read String.vi"("Name"=w382) -> ("String"=w381:string)  [unwired: 9 in, 1 out]
                n217 = Unbundle(w380) -> (w376:string[])
                n218 = Match First String(2:w376, 3:w381) -> (0:w377:i32)  [unwired: 1 out]
                n219 = property on="Test Ring" class="Ring (strict)"("Value"=w377, "Strings []"=w376) -> ()  [unwired: 2 in, 2 out]
                n220 = property on="Test Ring" class="Ring (strict)"("Visible"=TRUE) -> ()  [unwired: 2 in, 2 out]
                n221 = property on="Test Slider" class="Slide (strict)"("Visible"=FALSE) -> ()  [unwired: 2 in, 2 out]
              }
              frame "Exposure Priority  **" {
                n222 = Index Array(array=w388, index=3) -> (element=w389:cluster{string[]})
                n223 = call <vilib>:"NT Read String.vi"("Name"=w391) -> ("String"=w390:string)  [unwired: 9 in, 1 out]
                n224 = Unbundle(w389) -> (w385:string[])
                n225 = Match First String(2:w385, 3:w390) -> (0:w386:i32)  [unwired: 1 out]
                n226 = property on="Test Ring" class="Ring (strict)"("Value"=w386, "Strings []"=w385) -> ()  [unwired: 2 in, 2 out]
                n227 = property on="Test Ring" class="Ring (strict)"("Visible"=TRUE) -> ()  [unwired: 2 in, 2 out]
                n228 = property on="Test Slider" class="Slide (strict)"("Visible"=FALSE) -> ()  [unwired: 2 in, 2 out]
              }
              frame "Color Enable  **" {
                n229 = Index Array(array=w397, index=4) -> (element=w398:cluster{string[]})
                n230 = call <vilib>:"NT Read String.vi"("Name"=w400) -> ("String"=w399:string)  [unwired: 9 in, 1 out]
                n231 = Unbundle(w398) -> (w394:string[])
                n232 = Match First String(2:w394, 3:w399) -> (0:w395:i32)  [unwired: 1 out]
                n233 = property on="Test Ring" class="Ring (strict)"("Value"=w395, "Strings []"=w394) -> ()  [unwired: 2 in, 2 out]
                n234 = property on="Test Ring" class="Ring (strict)"("Visible"=TRUE) -> ()  [unwired: 2 in, 2 out]
                n235 = property on="Test Slider" class="Slide (strict)"("Visible"=FALSE) -> ()  [unwired: 2 in, 2 out]
              }
              frame Default {
                n236 = property on="Test Ring" class="Ring (strict)"("Visible"=FALSE) -> ()  [unwired: 2 in, 2 out]
                n237 = property on="Test Slider" class="Slide (strict)"("Visible"=FALSE) -> ()  [unwired: 2 in, 2 out]
              }
              frame "Brightness  **", "Color Level  **", "Compression  **", "FPS  **", "Sharpness  **" {
                n238 = call <vilib>:"NT Read Number.vi"("Name"=w406) -> ("Numeric"=w405:dbl)  [unwired: 9 in, 1 out]
                n239 = local write "Test Slider"(w405) -> ()
                n240 = property on="Test Slider" class="Slide (strict)"("Visible"=TRUE, "Scale.Maximum"=100.0 ("Scale.Range:Maximum")) -> ()  [unwired: 2 in, 2 out]
                n241 = property on="Test Ring" class="Ring (strict)"("Visible"=FALSE) -> ()  [unwired: 2 in, 2 out]
              }
            }
          }
        }
        n242 = property on="Progress" class="Clust (strict)"("Visible"=FALSE) -> ()  [unwired: 2 in, 2 out]
      }
      event "Test Name": Mouse Enter {
        # "Populate the ring with the list of tests"
        n243 = event-data() -> ()  [unwired: 1 in, 1 out]
        n244 = call <vilib>:"NT Read String Array.vi"("Name"="TestMode/TestList") -> ("String Array"=w414:string[])  [unwired: 9 in, 1 out]
        n245 = Build Array (concatenate)("Select the test to run...", w414) -> (w413:string[])
        n246 = property on="Test Name" class="Ring (strict)"("Strings []"=w413) -> ()  [unwired: 2 in, 2 out]
      }
      event "Test Name": Value Change {
        w416 = FALSE ("Visible")
        # "Tell the robot the test name to run"
        n247 = event-data() -> ("NewVal"=w420:u16)  [unwired: 1 in]
        n248 = property on="Test Name" class="Ring (strict)"() -> ("Strings []"=w421:string[])  [unwired: 2 in, 2 out]
        n249 = local write "Progress"(T11 {"Test Progress"=0, "Test Progress Text"=""} ("Progress")) -> ()
        n250 = Index Array(array=w421, index=w420) -> (element=w419:string)
        n251 = call <vilib>:"NT Write String.vi"("String"=w419, "Name"="TestMode/TestName") -> ()  [unwired: 9 in, 1 out]
        n252 = property on="Progress" class="Clust (strict)"("Visible"=TRUE) -> ()  [unwired: 2 in, 2 out]
        n253 = property on="Motor" class="Clust (strict)"("Visible"=w416) -> ()  [unwired: 2 in, 2 out]
        n254 = property on="Test Slider" class="Slide (strict)"("Visible"=w416) -> ()  [unwired: 2 in, 2 out]
        n255 = property on="On/Off" class="Bool (strict)"("Visible"=w416) -> ()  [unwired: 2 in, 2 out]
        n256 = property on="Rev/Fwd" class="Clust (strict)"("Visible"=w416) -> ()  [unwired: 2 in, 2 out]
        n257 = property on="Test Ring" class="Ring (strict)"("Visible"=w416) -> ()  [unwired: 2 in, 2 out]
      }
      event "Listbox": Double Click {
        n258 = event-data() -> ("PlatMods.Shift"=w424:bool, "Row"=w426:i32)  [unwired: 1 in]
        n259 = case shown="True" w424 {
          tunnel: w426 -> [w430 _]
          tunnel: 1 -> [w429 _]
          frame False {
            n260 = property on="Listbox" class="LstBox (strict)"() -> ("Item Symbols"=w428:i32[])  [unwired: 2 in, 2 out]
            n261 = Replace Array Subset(array=w428, new element=w429, index=w430) -> (w427:i32[])
            n262 = property on="Listbox" class="LstBox (strict)"("Item Symbols"=w427) -> ()  [unwired: 2 in, 2 out]
          }
          frame True {
            w431 = 0 ("Top Row")
            n263 = property on="Listbox" class="LstBox (strict)"() -> ("Number of Rows"=w433:u32)  [unwired: 2 in, 2 out]
            n264 = Initialize Array(0, w433) -> (w432:i32[])
            n265 = property on="Listbox" class="LstBox (strict)"("Top Row"=w431, "Value"=w431, "Item Symbols"=w432) -> ()  [unwired: 2 in, 2 out]
          }
        }
      }
      event "Listbox": Key Down {
        n266 = event-data() -> ("VKey"=w437:T24)  [unwired: 1 in]
        n267 = case shown="\"Left\", \"Right\"" w437 {
          selector: w437 -> [w442 _]
          tunnel: eventvkey."Left" ("VKey") -> [w440 _]
          frame "Left", "Right" {
            n268 = Equal?(x=w440, y=w442) -> (x = y?=w441:bool)
            n269 = Select(t=0, s=w441, f=1) -> (s? t:f=w443:i32)
            n270 = property on="Listbox" class="LstBox (strict)"() -> ("Item Symbols"=w446:i32[])  [unwired: 2 in, 2 out]
            n271 = Replace Array Subset(array=w446, new element=w443, index="Listbox") -> (w445:i32[])
            n272 = property on="Listbox" class="LstBox (strict)"("Item Symbols"=w445) -> ()  [unwired: 2 in, 2 out]
          }
          frame Default {
          }
        }
      }
      event "DB Camera Config": Value Change {
        n273 = event-data() -> ("NewVal"=w450:bool)  [unwired: 1 in]
        n274 = case shown="False" w450 {
          tunnel: w449 -> [w459 _]
          tunnel: [w452 w470] -> w448
          tunnel: w447 -> [w451 w470]
          frame False {
            w466 = "Camera"
            w469 = FALSE ("Visible")
            n275 = local read "Camera Settings"() -> (w458:T2)
            n276 = Index Array(array=w459) -> (element=w462:cluster{string[]})  [unwired: 1 in]
            n277 = Unbundle(w458) -> ("Frame Rate"=w457:i32, "Compression"=w456:i32, "Size"=w460:u16)
            n278 = Unbundle(w462) -> (w461:string[])
            n279 = Index Array(array=w461, index=w460) -> (element=w455:string)
            n280 = call-poly <vilib>:"Write Key.vi"("section"=w466, "value"=w455, "key"="Size", "refnum"=w451) -> ("refnum out"=w468:T23)  [unwired: 2 in, 5 out]
            n281 = call-poly <vilib>:"Write Key.vi"("section"=w466, "value"=w457, "key"="FrameRate", "refnum"=w468) -> ("refnum out"=w467:T23)  [unwired: 1 in, 6 out]
            n282 = local write "DB Camera Config"(w469) -> ()
            n283 = property on="Camera Settings" class="Clust (strict)"("Visible"=w469) -> ()  [unwired: 2 in, 2 out]
            n284 = call-poly <vilib>:"Write Key.vi"("section"=w466, "value"=w456, "key"="Compression", "refnum"=w467) -> ("refnum out"=w453:T23)  [unwired: 1 in, 6 out]
            n285 = call <vilib>:"Close Config Data.vi"("refnum"=w453) -> ("file path"=w454:path)  [unwired: 2 in, 8 out]
            n286 = call <vilib>:"Open Config Data.vi"("configuration file path"=w454) -> ("refnum"=w452:T23)  [unwired: 8 in, 2 out]
          }
          frame True {
            n287 = property on="Camera Settings" class="Clust (strict)"("Visible"=TRUE) -> ()  [unwired: 2 in, 2 out]
          }
        }
      }
      event "Camera Settings": Value Change {
        n288 = event-data() -> ("NewVal"=w483:T2)  [unwired: 1 in]
        n289 = Index Array(array=w479) -> (element=w478:cluster{string[]})  [unwired: 1 in]
        n290 = Unbundle(w483) -> ("Frame Rate"=w474:i32, "Compression"=w473:i32, "Size"=w476:u16)
        n291 = Unbundle(w478) -> (w477:string[])
        n292 = Index Array(array=w477, index=w476) -> (element=w475:string)
        n293 = Format Into String(format string="%s   %dfps   %d%%", w475, w474, w473) -> (resulting string=w480:string)  [unwired: 2 in, 1 out]
        n294 = Build Array(w480) -> (w481:string[])
        n295 = property on="DB Camera Config" class="Bool (strict)"("Strings [4]"=w481) -> ()  [unwired: 2 in, 2 out]
      }
      event "Motor.Enable": Value Change {
        n296 = event-data() -> ("NewVal"=w489:bool)  [unwired: 1 in]
        n297 = Unbundle("Motor") -> ("Value"=w488:dbl)  [unwired: 1 out]
        n298 = Select(t=w488, s=w489, f=0.0) -> (s? t:f=w486:dbl)
        n299 = call <vilib>:"NT Write Number.vi"("Numeric"=w486, "Name"=w485) -> ()  [unwired: 9 in, 1 out]
      }
      event "Test Slider": Value Change {
        n300 = event-data() -> ("NewVal"=w492:dbl)  [unwired: 1 in]
        n301 = call <vilib>:"NT Write Number.vi"("Numeric"=w492, "Name"=w493) -> ()  [unwired: 9 in, 1 out]
      }
      event "On/Off": Value Change {
        n302 = event-data() -> ("NewVal"=w497:bool)  [unwired: 1 in]
        n303 = Boolean To (0,1)(Boolean=w497) -> (0, 1=w496:i16)
        n304 = call <vilib>:"NT Write Number.vi"("Numeric"=w496, "Name"=w495) -> ()  [unwired: 9 in, 1 out]
      }
      event "Rev/Fwd": Value Change {
        n305 = event-data() -> ("NewVal.Forward"=w505:bool, "NewVal.Reverse"=w504:bool)  [unwired: 1 in]
        n306 = Boolean To (0,1)(Boolean=w505) -> (0, 1=w501:i16)
        n307 = Boolean To (0,1)(Boolean=w504) -> (0, 1=w503:i16)
        n308 = Negate(x=w503) -> (-x=w502:i16)
        n309 = Add(x=w501, y=w502) -> (x+y=w500:i16)
        n310 = call <vilib>:"NT Write Number.vi"("Numeric"=w500, "Name"=w499) -> ()  [unwired: 9 in, 1 out]
      }
      event "Test Ring": Value Change {
        n311 = event-data() -> ("NewVal"=w509:u16)  [unwired: 1 in]
        n312 = property on="Test Ring" class="Ring (strict)"() -> ("Strings []"=w510:string[])  [unwired: 2 in, 2 out]
        n313 = Index Array(array=w510, index=w509) -> (element=w508:string)
        n314 = call <vilib>:"NT Write String.vi"("String"=w508, "Name"=w507) -> ()  [unwired: 9 in, 1 out]
      }
      event "Rec Mode": Value Change {
        # "Update globals for recording mode and path to read log from.\nClear when logging and let NetworkTables set path for vision to\nuse."
        n315 = event-data() -> ("NewVal"=w520:enum32{"Stop", "Record", "Playback"})  [unwired: 1 in]
        n316 = global write "WPI_DashboardLogging Global.vi" "Logging Filename"(path "") -> ()
        n317 = global write "WPI_DashboardLogging Global.vi" "Recording"(w520) -> ()
        n318 = case shown="\"Stop\", \"Record\"" w520 {
          tunnel: w519 -> [_ w522 w530]
          tunnel: [_ _ w529] -> w516
          tunnel: [_ _ w528] -> _
          tunnel: w514 -> [_ _ w526]
          tunnel: cluster{i32, i32} {-250, 170} -> [_ _ w525]
          tunnel: [_ _ T25 {"Image Size"=TRUE, "Image Type"=TRUE, "Pixel Value"=TRUE, "ROI Information"=TRUE, "Zoom Factor"=FALSE} ("Image Information Shown:All Elements")] -> w512
          tunnel: [_ _ TRUE ("Zoom Factor")] -> w511
          frame Default {
          }
          frame "Stop", "Record" {
            # "Place Window too"
            n319 = invoke class="VI" method="FP.Close"(reference=w522) -> (reference out=w521:refnum<vi>)  [unwired: 2 in, 2 out]
            n320 = invoke class="VI" method="Abort VI"(reference=w521) -> ()  [unwired: 2 in, 3 out]
          }
          frame "Playback" {
            n321 = call "Open Playback Panel.vi"("Offset"=w525, "DB VI Ref"=w526, "Playback in"=w530) -> ("Playback out"=w527:refnum<vi>)  [unwired: 8 in]
            n322 = register-events(w527) -> (reference out=w529:refnum<event-registration>, error out=w528:errorcluster)  [unwired: 2 in]
          }
        }
        n323 = property on="Camera Image" class="ImageControl"("Image Information Shown"=w512, "Image Information Visible"=w511) -> ()  [unwired: 2 in, 2 out]
        n324 = call <vilib>:"WPI_DashboardNT Log FieldName Cache.vi"("Operation"=enum16{"Lookup/Add", "Index", "Clear"}."Clear") -> ()  [unwired: 8 in, 3 out]
      }
      event Panel Close {
        w531 = enum32{"Stop", "Record", "Playback"}."Stop" ("Rec Mode")
        n325 = event-data() -> ()  [unwired: 1 in, 4 out]
        n326 = local write "Rec Mode"(w531) -> ()
        n327 = global write "WPI_DashboardLogging Global.vi" "Recording"(w531) -> ()
      }
      event Panel Close {
        # "Abort playback window and ourself"
        n328 = event-data() -> ()  [unwired: 1 in, 4 out]
        n329 = invoke class="VI" method="FP.Close"(reference=w536) -> (reference out=w535:refnum<vi>)  [unwired: 2 in, 2 out]
        n330 = invoke class="VI" method="Abort VI"(reference=w535) -> (error out=w534:errorcluster)  [unwired: 2 in, 2 out]
        n331 = invoke class="VI" method="Abort VI"(error in=w534) -> ()  [unwired: 2 in, 3 out]
      }
    }
  }
  n332 = property on="On/Off" class="Bool (strict)"("Visible"=w25) -> ()  [unwired: 2 in, 2 out]
  n333 = property on="Motor" class="Clust (strict)"("Visible"=w25) -> ()  [unwired: 2 in, 2 out]
  n334 = property on="Progress" class="Clust (strict)"("Visible"=w25) -> ()  [unwired: 2 in, 2 out]
  n335 = property on="Test Ring" class="Ring (strict)"("Visible"=w25) -> ()  [unwired: 2 in, 2 out]
  n336 = property on="Rev/Fwd" class="Clust (strict)"("Visible"=w25) -> ()  [unwired: 2 in, 2 out]
  n337 = local write "DB Camera Config"(w25) -> ()
  n338 = property on="Camera Settings" class="Clust (strict)"("Visible"=w25) -> ()  [unwired: 2 in, 2 out]
  n339 = global write "WPI_DashboardLogging Global.vi" "Recording"(w8) -> ()
  n340 = local write "Rec Mode"(w8) -> ()
